vi "confirm hardware config.vi"() -> ()   [LabVIEW 2012]
doc: "SciScan 1.2 160622"
uses:
  GFG/GFGstringGet.vi
  GFG/GFG library.lvlib
  <vilib>/nisyscfg/nisyscfg.lvlib
  <resource>/objmgr/nisysapi.rc
panel:
  out "error out":errorcluster
  in  "FPGA device name":u16(ring)
  in  "stop":bool
  in  "FPGA model":u16(ring) items=["PXIe7962R", "PXIe7961R"]
  in  "digitizer model":u16(ring) items=["NI5751", "NI5734"]
  in  "AO card model":u16(ring) items=["PXI6259", "PXIe6341"]
  # "Configure Resonant hardware"
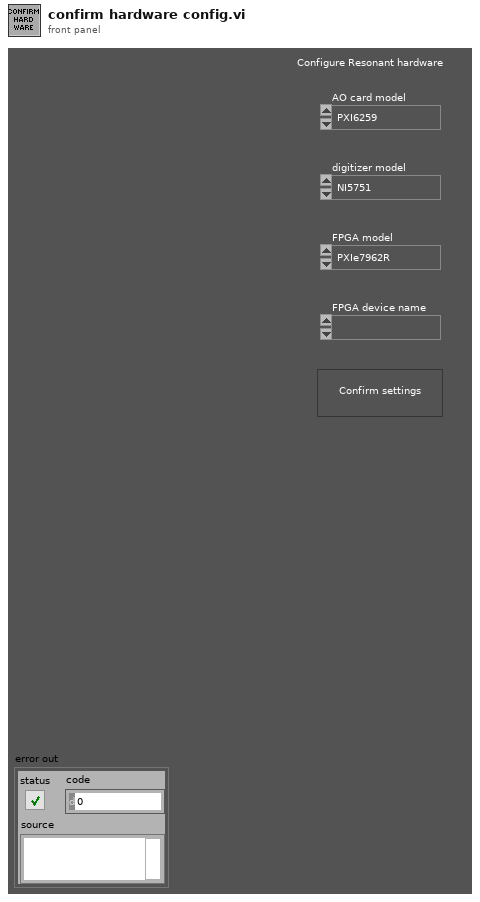
[diagram p1: front panel]
types:
  T1 = enum8{"Enabled", "Disabled", "Disabled and Grayed Out"}
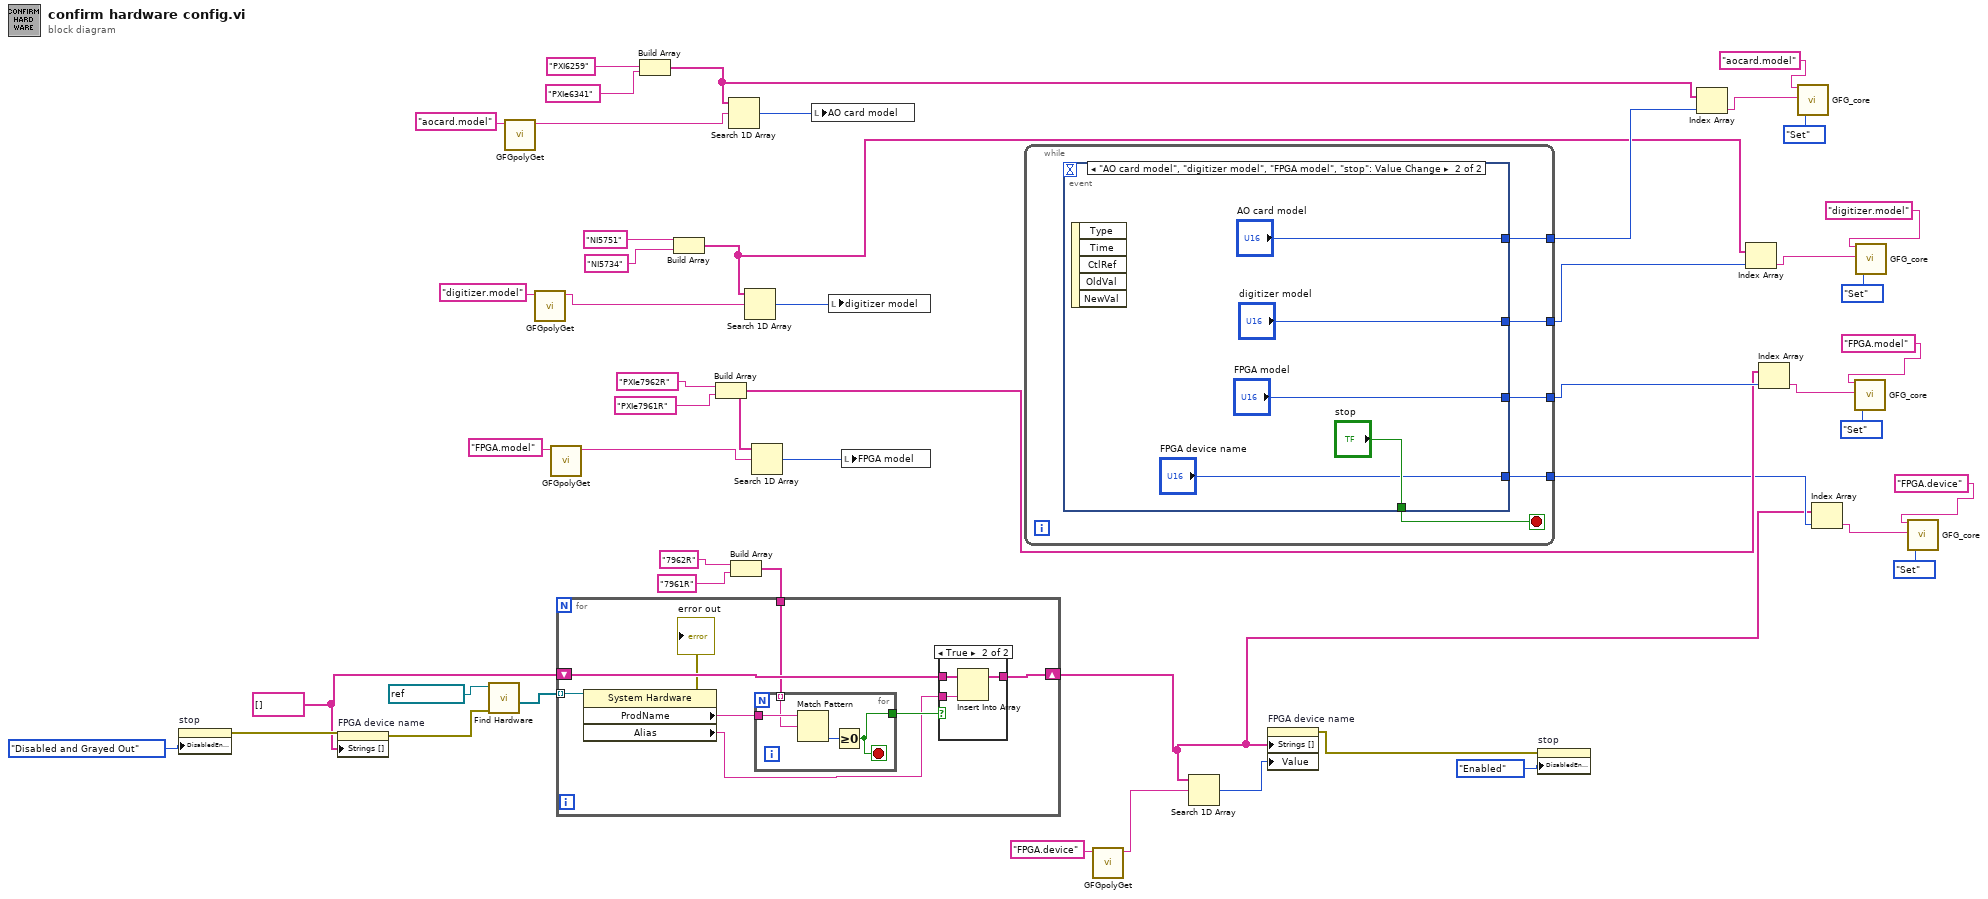
[diagram p0: block diagram]
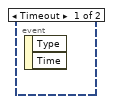
[diagram p3: hidden frame]
diagram:
  w2 = string[] []
  n1 = property on="stop" class="Bool"("DisabledEnum"=T1."Disabled and Grayed Out" ("Disabled")) -> (error out=w16:errorcluster)  [unwired: 2 in, 1 out]
  n2 = property on="FPGA device name" class="Ring (strict)"(error in=w16, "Strings []"=w2) -> (error out=w3:errorcluster)  [unwired: 1 in, 1 out]
  n3 = call <vilib>:"Find Hardware.vi"("error in (no error)"=w3, "Session in"=refnum<k21> "localhost" ("Session in (localhost)")) -> ("Resources out"=w7:refnum<k20>[])  [unwired: 6 in, 3 out]
  n4 = call-poly "GFGpolyGet.vi"("Variable Name in"="aocard.model") -> ("String"=w40:string)  [unwired: 9 in, 1 out]
  n5 = call-poly "GFGpolyGet.vi"("Variable Name in"="digitizer.model") -> ("String"=w37:string)  [unwired: 9 in, 1 out]
  n6 = call-poly "GFGpolyGet.vi"("Variable Name in"="FPGA.model") -> ("String"=w35:string)  [unwired: 9 in, 1 out]
  n7 = Build Array("PXI6259", "PXIe6341") -> (w31:string[])
  n8 = Build Array("NI5751", "NI5734") -> (w30:string[])
  n9 = Build Array("PXIe7962R", "PXIe7961R") -> (w29:string[])
  n10 = Search 1D Array(1D array=w31, element=w40) -> (index of element=w39:i32)  [unwired: 1 in]
  n11 = Build Array("7962R", "7961R") -> (w4:string[])
  n12 = for {
    tunnel: w7 -> [w57] mode=indexing
    shift-right: [w54] -> w1
    shift-left: w2 -> [w55]
    tunnel: w4 -> [w50]
    n13 = property class="System Hardware"(reference=w57) -> (error out=→"error out":errorcluster, "ProdName"=w52:string, "Alias"=w53:string)  [unwired: 1 in, 1 out]
    n14 = for {
      tunnel: [w58] -> w56
      tunnel: w52 -> [w60]
      tunnel: w50 -> [w59] mode=indexing
      stop <- w58 stop-if-true
      n15 = Match Pattern(string=w60, regular expression=w59) -> (offset past match=w61:i32)  [unwired: 1 in, 3 out]
      n16 = Greater Or Equal To 0?(x=w61) -> (x >= 0?=w58:bool)
    }
    n17 = case shown="True" w56 {
      tunnel: w55 -> [w62 w65]
      tunnel: w53 -> [_ w64]
      tunnel: [w62 w63] -> w54
      frame False {
      }
      frame True {
        n18 = Insert Into Array(array=w65, new element=w64) -> (w63:string[])  [unwired: 1 in]
      }
    }
  }
  n19 = Search 1D Array(1D array=w30, element=w37) -> (index of element=w38:i32)  [unwired: 1 in]
  n20 = Search 1D Array(1D array=w29, element=w35) -> (index of element=w36:i32)  [unwired: 1 in]
  n21 = local write "AO card model"(w39) -> ()
  n22 = local write "digitizer model"(w38) -> ()
  n23 = local write "FPGA model"(w36) -> ()
  n24 = while {
    tunnel: [w69] -> w34
    tunnel: [w68] -> w33
    tunnel: [w67] -> w32
    tunnel: [w66] -> w9
    stop <- w70 stop-if-true
    n25 = event shown="[1] \"AO card model\", \"digitizer model\", \"FPGA model\", \"stop\": Value Change" {
      selector: _ -> [_ _]
      dyn-events: _ -> [_ _]
      timeout: _ -> [_ _]
      tunnel: [_ "stop"] -> w70
      tunnel: [_ "AO card model"] -> w69
      tunnel: [_ "digitizer model"] -> w68
      tunnel: [_ "FPGA model"] -> w67
      tunnel: [_ "FPGA device name"] -> w66
      event Timeout {
        n26 = event-data() -> ()  [unwired: 1 in, 2 out]
      }
      event "AO card model", "digitizer model", "FPGA model", "stop": Value Change {
        n27 = event-data() -> ()  [unwired: 1 in, 5 out]
      }
    }
  }
  n28 = call-poly "GFGpolyGet.vi"("Variable Name in"="FPGA.device") -> ("String"=w18:string)  [unwired: 9 in, 1 out]
  n29 = Search 1D Array(1D array=w1, element=w18) -> (index of element=w17:i32)  [unwired: 1 in]
  n30 = property on="FPGA device name" class="Ring (strict)"("Strings []"=w1, "Value"=w17) -> (error out=w13:errorcluster)  [unwired: 2 in, 1 out]
  n31 = property on="stop" class="Bool"(error in=w13, "DisabledEnum"=T1."Enabled" ("Disabled")) -> ()  [unwired: 1 in, 2 out]
  n32 = Index Array(array=w31, index=w34) -> (element=w27:string)
  n33 = Index Array(array=w30, index=w33) -> (element=w24:string)
  n34 = Index Array(array=w29, index=w32) -> (element=w21:string)
  n35 = call "GFG_core.vi"("Variable Name in"="aocard.model", "Variant in"=w27, "Action"=enum16{"Init", "Set", "Get", "Clear"}."Set") -> ()  [unwired: 10 in, 7 out]
  n36 = Index Array(array=w1, index=w9) -> (element=w11:string)
  n37 = call "GFG_core.vi"("Variable Name in"="FPGA.model", "Variant in"=w21, "Action"=enum16{"Init", "Set", "Get", "Clear"}."Set") -> ()  [unwired: 10 in, 7 out]
  n38 = call "GFG_core.vi"("Variable Name in"="digitizer.model", "Variant in"=w24, "Action"=enum16{"Init", "Set", "Get", "Clear"}."Set") -> ()  [unwired: 10 in, 7 out]
  n39 = call "GFG_core.vi"("Variable Name in"="FPGA.device", "Variant in"=w11, "Action"=enum16{"Init", "Set", "Get", "Clear"}."Set") -> ()  [unwired: 10 in, 7 out]
